vi "pmu_Analog Digit Scale CFG-3.vi"(6 "nominal frequency":enum16{"50 Hz", "60 Hz"}(ring), 7 "analog scaling":T1, 8 "dfreq in":sgl, 9 "freq in":sgl, 10 "analogs in":sgl[](array[numeric]), 11 "format":u16) -> (0 "freq out of range":bool, 1 "analog out of range":bool, 2 "analogs byte array":u8[](array[numeric]), 3 "dfreq byte array":u8[](array[numeric]), 4 "df/dt out of range":bool, 5 "freq byte array":u8[](array[numeric]))   [LabVIEW 2014, in "NI_EP_PMU.lvlib"]
uses:
  <vilib>/addons/Electrical Power/PMU/NI_EP_PMU.lvlib
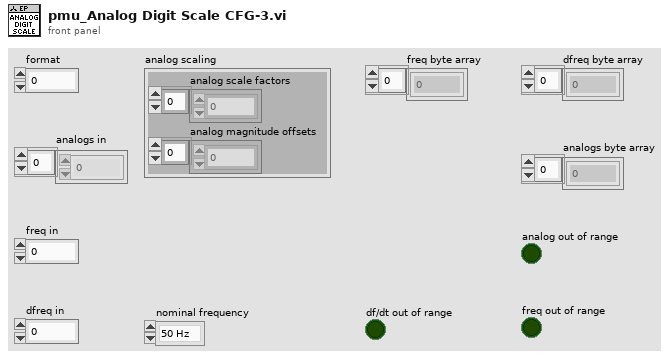
[diagram p1: front panel]
types:
  T1 = cluster{"analog scale factors":sgl[], "analog magnitude offsets":sgl[]}
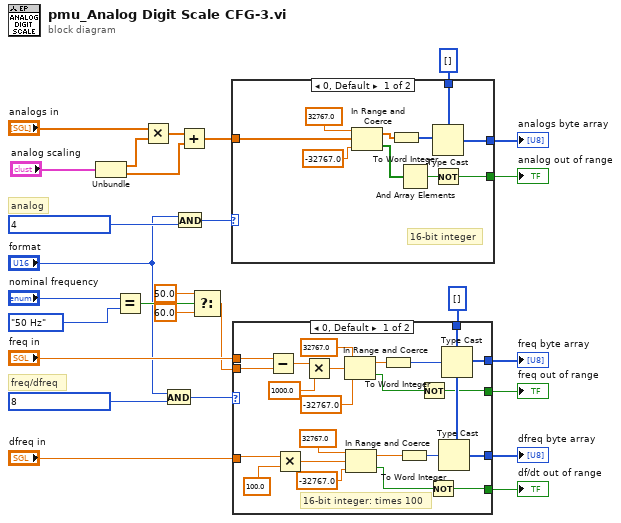
[diagram p0: block diagram]
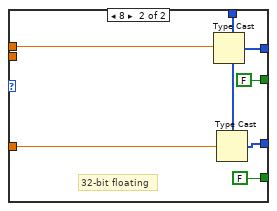
[diagram p2: hidden frame]
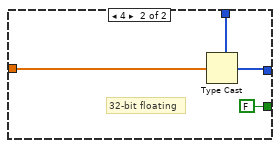
[diagram p3: hidden frame]
diagram:
  # "freq/dfreq"
  # "analog"
  n1 = Unbundle("analog scaling") -> ("analog scale factors"=w4:sgl[], "analog magnitude offsets"=w2:sgl[])
  n2 = Equal?(x="nominal frequency", y=enum16{"50 Hz", "60 Hz"}."50 Hz" ("nominal frequency 2")) -> (x = y?=w14:bool)
  n3 = Multiply(x="analogs in", y=w4) -> (x*y=w3:sgl[])
  n4 = And(x="format", y=u16 8 ("x")) -> (x .and. y?=w24:u16)
  n5 = And(x="format", y=u16 4 ("x")) -> (x .and. y?=w25:u16)
  n6 = Add(x=w3, y=w2) -> (x+y=w1:sgl[])
  n7 = Select(t=50.0, s=w14, f=60.0) -> (s? t:f=w11:dbl)
  n8 = case shown="0, Default" w25 {
    tunnel: w1 -> [w32 w40]
    tunnel: u8[] [] ("appended array") -> [w36 w41]
    tunnel: [w35 w39] -> w22
    tunnel: [w28 FALSE] -> w8
    frame 0, Default {
      # "16-bit integer"
      n9 = In Range and Coerce(upper limit=sgl 32767.0 ("y"), x=w32, lower limit=sgl -32767.0 ("y")) -> (coerced(x)=w31:sgl[], In Range?=w29:bool[])
      n10 = To Word Integer(number=w31) -> (16bit integer=w37:i16[])
      n11 = And Array Elements(Boolean array=w29) -> (logical AND=w30:bool)
      n12 = Type Cast(type=w36, x=w37) -> (*(type *) &x=w35:u8[])
      n13 = Not(x=w30) -> (.not. x?=w28:bool)
    }
    frame 4 {
      # "32-bit floating"
      n14 = Type Cast(type=w41, x=w40) -> (*(type *) &x=w39:u8[])
    }
  }
  "analogs byte array" <- w22
  "analog out of range" <- w8
  n15 = case shown="0, Default" w24 {
    tunnel: "freq in" -> [w60 w68]
    tunnel: "dfreq in" -> [w48 w65]
    tunnel: u8[] [] ("appended array") -> [w63 w70]
    tunnel: [w64 w71] -> w18
    tunnel: [w61 w69] -> w17
    tunnel: w11 -> [w59 _]
    tunnel: [w44 FALSE] -> w10
    tunnel: [w43 FALSE] -> w9
    frame 0, Default {
      # "16-bit integer: times 100"
      n16 = Subtract(x=w60, y=w59) -> (x-y=w58:dbl)
      n17 = Multiply(x=w48, y=sgl 100.0) -> (x*y=w46:sgl)
      n18 = Multiply(x=w58, y=1000.0) -> (x*y=w56:dbl)
      n19 = In Range and Coerce(upper limit=32767.0 ("y"), x=w56, lower limit=-32767.0 ("y")) -> (coerced(x)=w53:dbl, In Range?=w45:bool)
      n20 = In Range and Coerce(upper limit=sgl 32767.0 ("y"), x=w46, lower limit=sgl -32767.0 ("y")) -> (coerced(x)=w49:sgl, In Range?=w42:bool)
      n21 = To Word Integer(number=w53) -> (16bit integer=w52:i16)
      n22 = To Word Integer(number=w49) -> (16bit integer=w62:i16)
      n23 = Not(x=w45) -> (.not. x?=w44:bool)
      n24 = Not(x=w42) -> (.not. x?=w43:bool)
      n25 = Type Cast(type=w63, x=w62) -> (*(type *) &x=w61:u8[])
      n26 = Type Cast(type=w63, x=w52) -> (*(type *) &x=w64:u8[])
    }
    frame 8 {
      # "32-bit floating"
      n27 = Type Cast(type=w70, x=w68) -> (*(type *) &x=w71:u8[])
      n28 = Type Cast(type=w70, x=w65) -> (*(type *) &x=w69:u8[])
    }
  }
  "freq byte array" <- w18
  "dfreq byte array" <- w17
  "freq out of range" <- w10
  "df/dt out of range" <- w9
